vi "Load Core Sequential.vi"(0 "Class Loader in":refnum<class "Class Loader.lvclass">, 5 "Caller Enqueuer":refnum<class "Message Enqueuer.lvclass">, 7 "Reference Class Path":path, 9 "Class Relative Paths Path":path, 11 "error in (no error)":errorcluster) -> (4 "Class Loader out":refnum<class "Class Loader.lvclass">, 15 "error out":errorcluster)   [LabVIEW 2023, in "Class Loader.lvlib" / "Class Loader.lvclass"]
uses:
  Class Loader.lvclass
  <vilib>/ActorFramework/Message Enqueuer/Message Enqueuer.lvclass
  Class Loader.lvclass/Class Loader.ctl
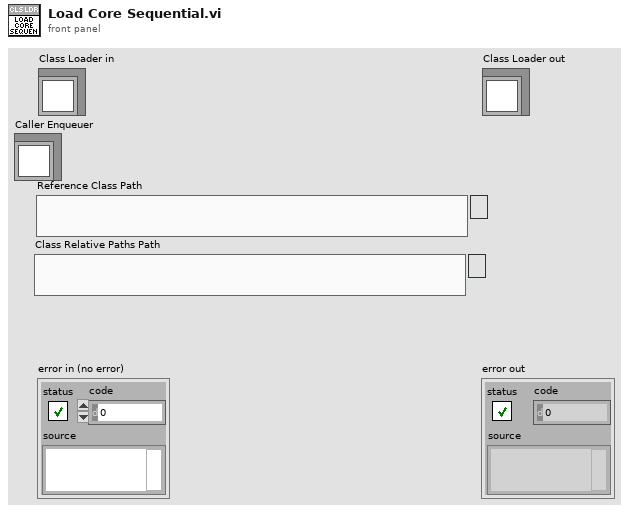
[diagram p1: front panel]
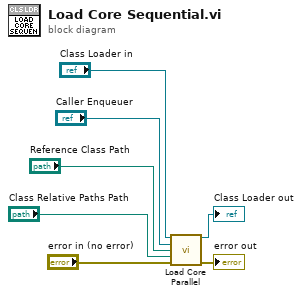
[diagram p0: block diagram]
diagram:
  n1 = call "Load Core Parallel.vi"("Class Loader in"="Class Loader in", "Caller Enqueuer"="Caller Enqueuer", "Reference Class Path"="Reference Class Path", "Class Relative Paths Path"="Class Relative Paths Path", "error in (no error)"="error in (no error)") -> ("Class Loader out"=→"Class Loader out":refnum<class "Class Loader.lvclass">, "error out"=→"error out":errorcluster)  [unwired: 9 in]
